vi "Get RegistrationRequest.vi"(8 "error in (no error)":errorcluster, 11 "gRPCid":T2) -> (0 "error out":errorcluster, 2 "Request Data":T1, 3 "gRPCid out":T2)   [LabVIEW 2019, in "OOP Server.lvclass"]
uses:
  OOP Server.lvclass
  gRPC interface/Server API/typeDefs/grpcId.ctl
  RegistrationRequest_Data.ctl
  905457ba-43ee-4d7e-b70e-0cf7ac2d3d08.vi
  gRPC interface/gprc-lvsupport.lvlib
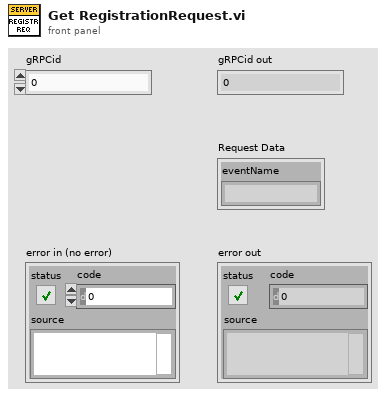
[diagram p1: front panel]
types:
  T1 = typedef "OOP Server.lvclass/RegistrationRequest_Data.ctl" = cluster{"eventName":string}
  T2 = typedef "gprc-lvsupport.lvlib/grpcId.ctl" = u64
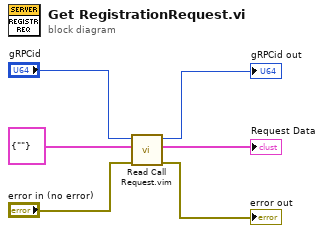
[diagram p0: block diagram]
diagram:
  n1 = call "Read Call Request.vim"("error in (no error)"="error in (no error)", "Data Type"=T1 {"eventName"=""} ("RegistrationRequest_Data"), "gRPCid in"="gRPCid") -> ("error out"=→"error out":errorcluster, "Request Data"=→"Request Data":T1, "gRPCid out"=→"gRPCid out":T2)  [unwired: 6 in]
